vi "_006.vi"() -> ()   [LabVIEW 2024]
panel:
  out "Borrow":bool
  out "Difference":bool
  in  "B in":bool
  in  "B":bool
  in  "A":bool
  out "Borrow :":bool
  out "Difference :":bool
  in  "B":bool
  in  "A":bool
  # "Subtractors :"
  # "Half Subtractor ( Truth Table ) :"
  # "Inputs   Outputs \nA  B   Diff   Borrow \n0  0  -> 0       0 \n0  1   -> 1        1\n1   0  -> 1        0\n1   1   -> 0       0"
  # "Full Subtractor ( Truth Table ) :"
  # "Inputs      Outputs      \nA  B  B in   Diff    Bout \n0  0   0  ->  0       0 \n0  0   1   ->  1        1\n0  1    0  ->  1        1\n0  1    1   ->  0       1\n1   0   0  ->  1        0\n1   0   1   ->  0       0\n1   1    0  ->  0       0\n1   1    1   ->  1        1"
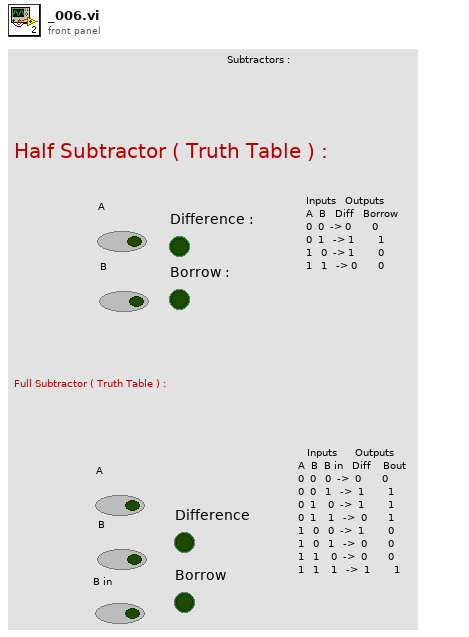
[diagram p1: front panel]
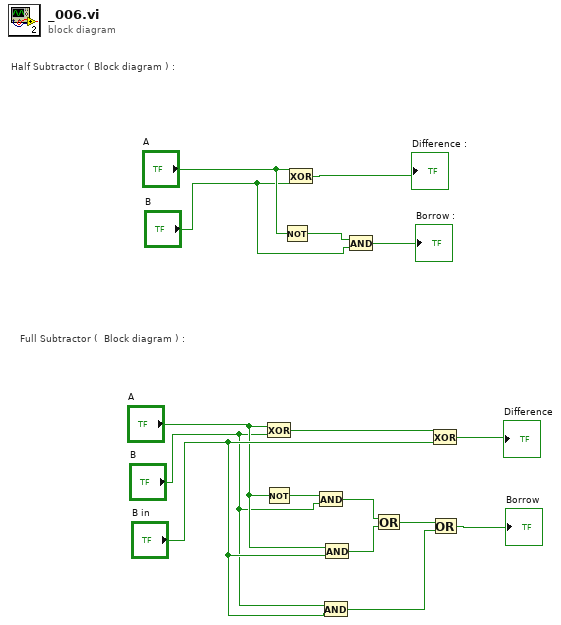
[diagram p0: block diagram]
diagram:
  # "Full Subtractor (  Block diagram ) :"
  # "Half Subtractor ( Block diagram ) :"
  n1 = Exclusive Or(1:"B", 2:"A") -> (0:w11:bool)
  n2 = Not(x="A") -> (.not. x?=w10:bool)
  n3 = Not(x="A") -> (.not. x?=w15:bool)
  n4 = Exclusive Or(1:"B", 2:"A") -> (0:→"Difference :":bool)
  n5 = And(x=w10, y="B") -> (x .and. y?=w6:bool)
  n6 = And(x="B", y="B in") -> (x .and. y?=w4:bool)
  n7 = And(x="A", y="B in") -> (x .and. y?=w5:bool)
  n8 = And(x=w15, y="B") -> (x .and. y?=→"Borrow :":bool)
  n9 = Or(x=w6, y=w5) -> (x .or. y?=w3:bool)
  n10 = Exclusive Or(1:"B in", 2:w11) -> (0:→"Difference":bool)
  n11 = Or(x=w3, y=w4) -> (x .or. y?=→"Borrow":bool)
